vi "ADB-BlueTooth_2.vi"(11 "COM Port":refnum<visa-resource-name>="COM18") -> (0 "error out":errorcluster, 1 "Connectet":bool, 2 "AT CMD\n Status":bool, 3 "ADB PID":string, 4 "RSSI":i32)   [LabVIEW 2018]
panel:
  out "Progres Bar":u8(slide) scale=0.0..10.0
  out "ADB Data Monitor":string
  out "connect str1":string
  out "connect str2":string
  out "BLE-NINA-B1":string
  out "Mgg":string
  out "AT Cmd INI":string[][](array[string])=[["AT+CPWROFF", "", "+STARTUP"], ["AT+GMI", "u-blox", "OK"], ["AT+GMM", "NINA-B1", "OK"], ["ATI9", "NINA-B11X-5.0.0-011-0", "OK"], ["AT+GMR", "5.0.0-011", "OK"], ["AT+UMLA=1", "+UMLA:CCF95792B245", "OK"], ["AT+UBTLE=1", "", "OK"], ["AT&W", "", "OK"], ["AT+CPWROFF", "", "OK"], ["+AT+UBTLE?", "+UBTLE:1", "OK"]]
  out "AT-CMD/Date Monitor":string="\r\n"
  out "Status":T1(ring)
  out "Name":string
  out "SRS":string
  # "ADB-BlueTooth TEST"
  # "dbm"
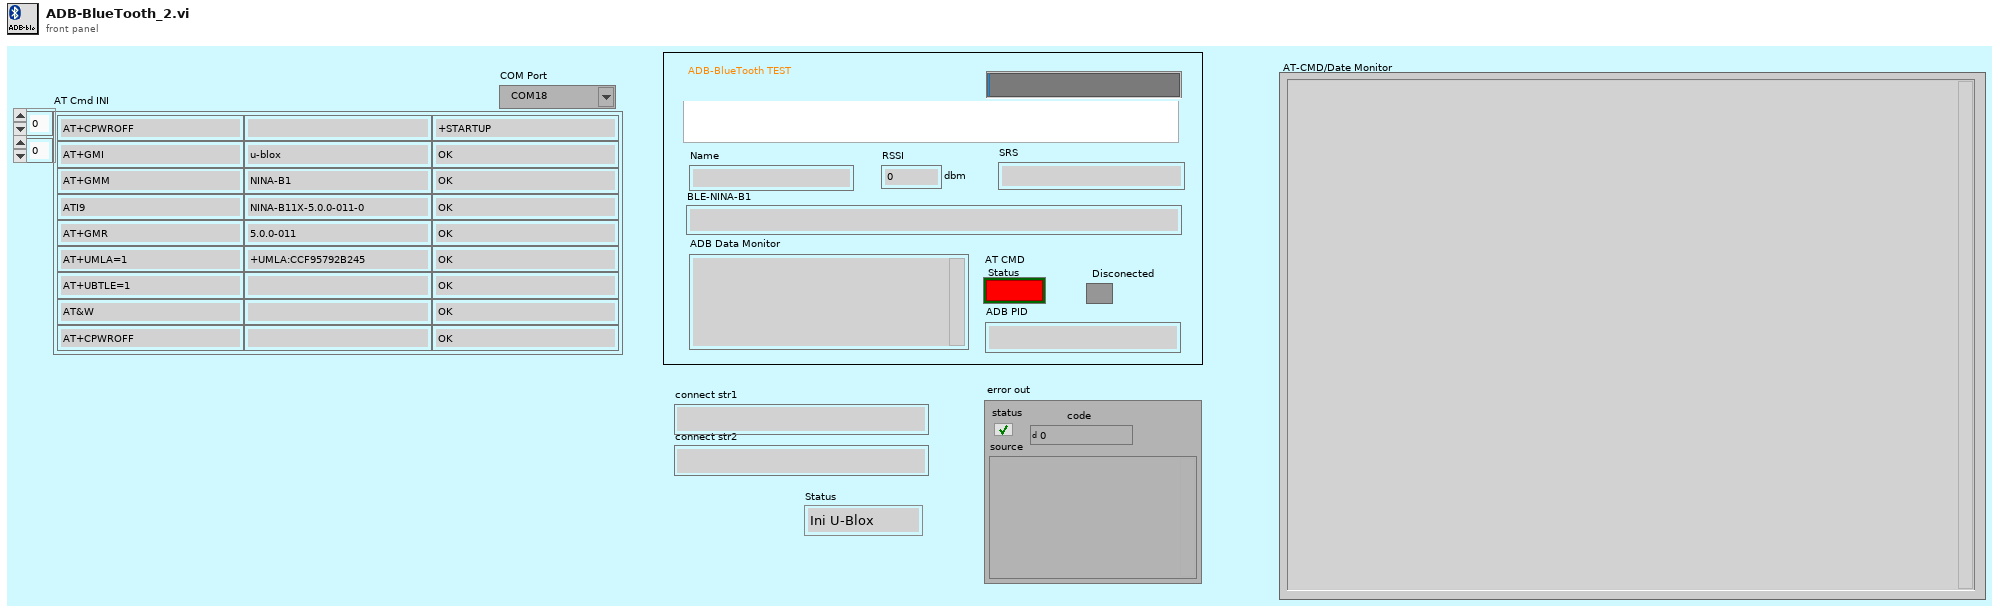
[diagram p1: front panel]
types:
  T1 = enum16{"Ini U-Blox", "Scan BLE Dev", "Connect to BLE", "Go-To DATA Mode", "Set BLE Admin", "BLE Red PID", "QUIT PAS/FALSE", "QUIT Err"}
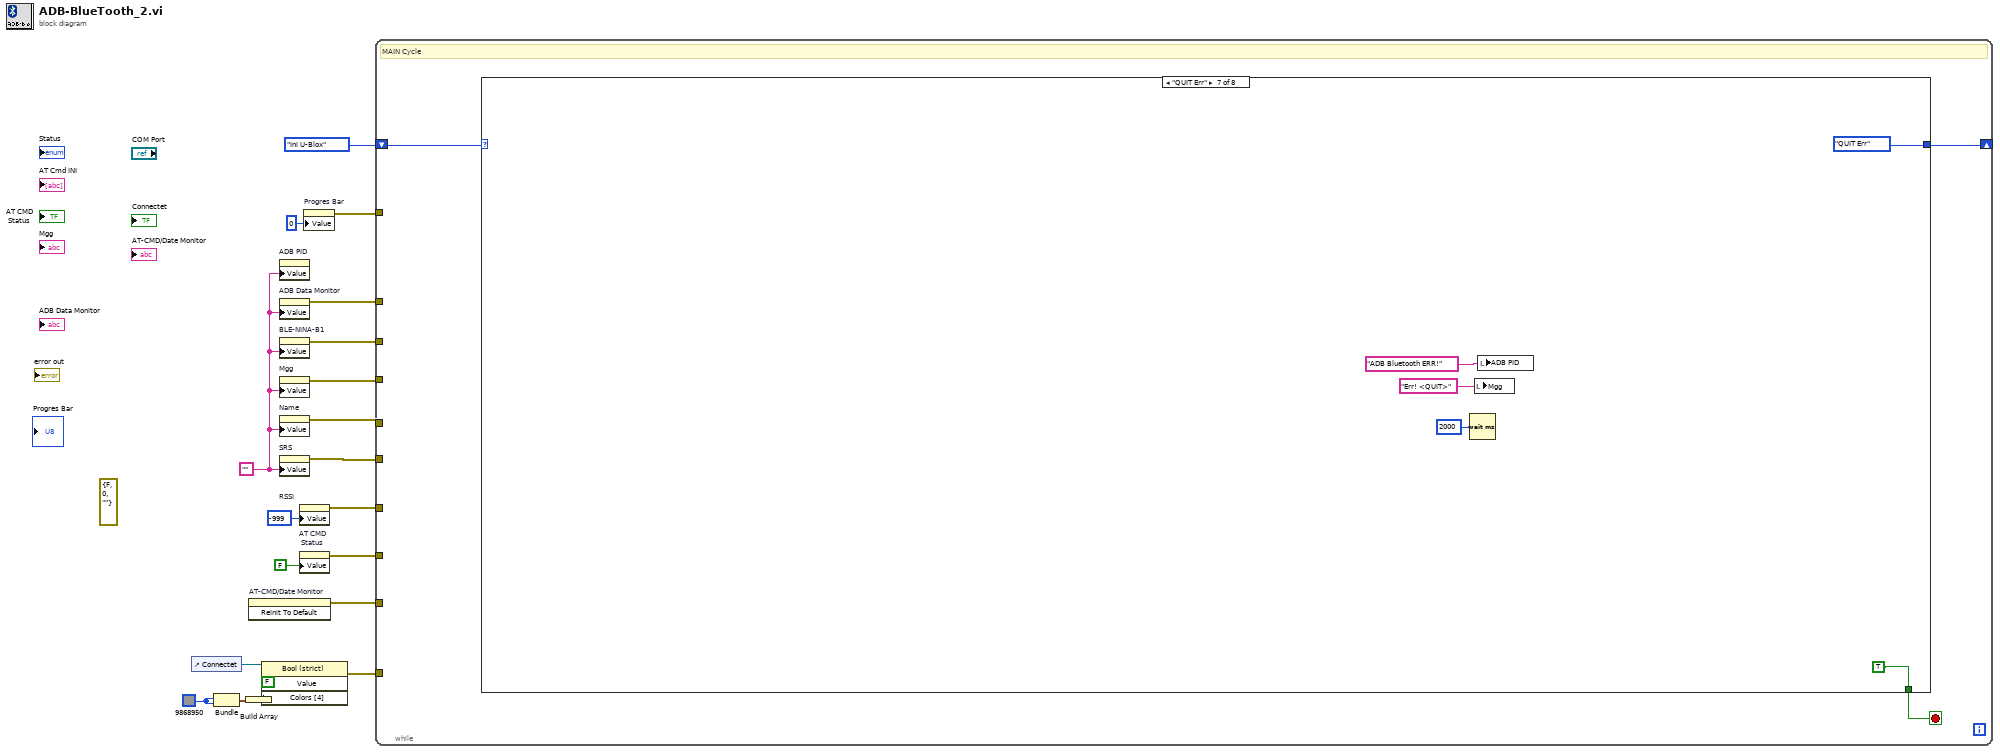
[diagram p0: block diagram]
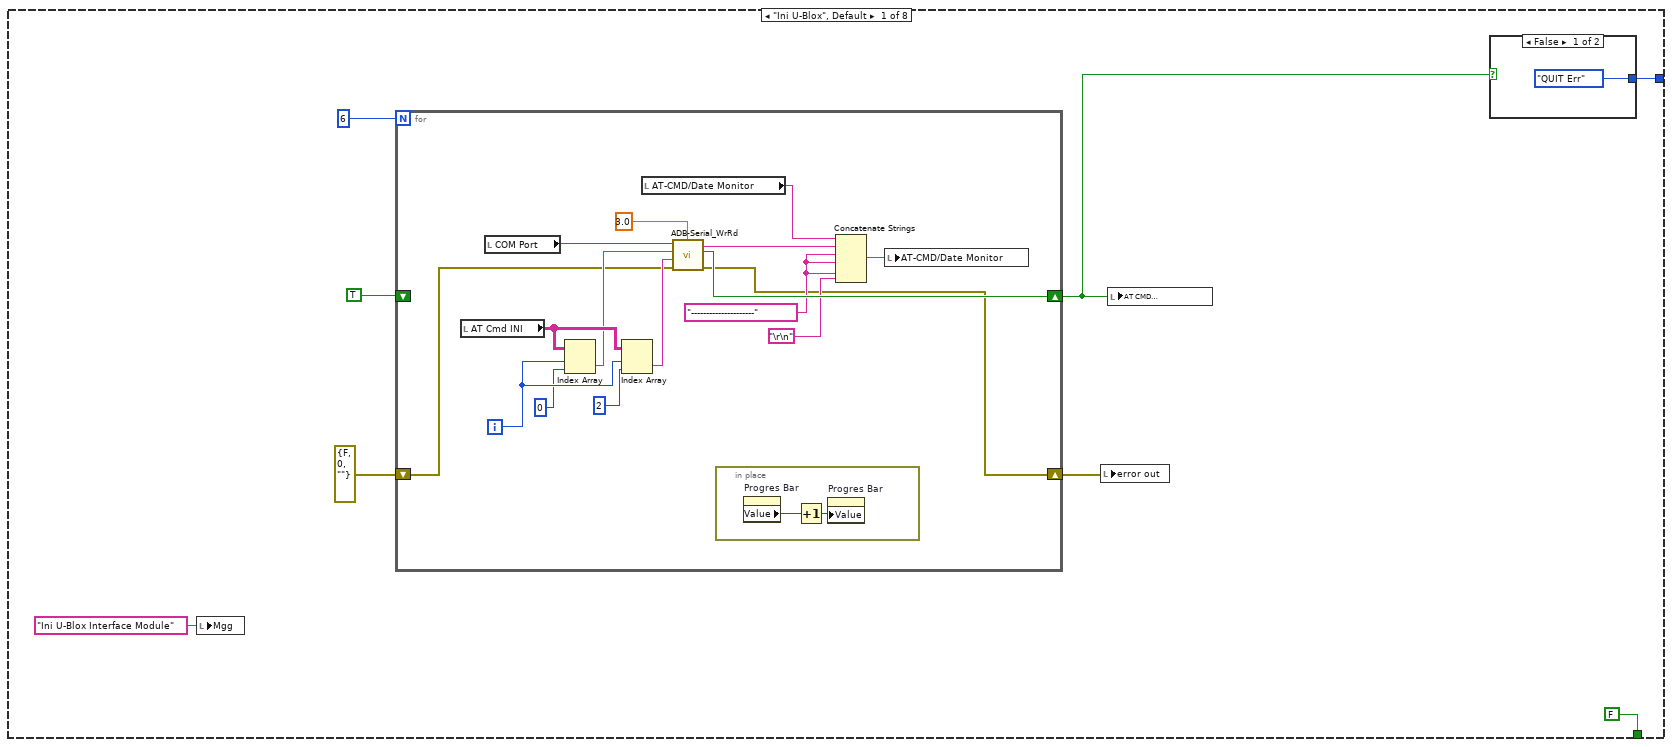
[diagram p2: hidden frame]
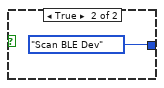
[diagram p3: hidden frame]
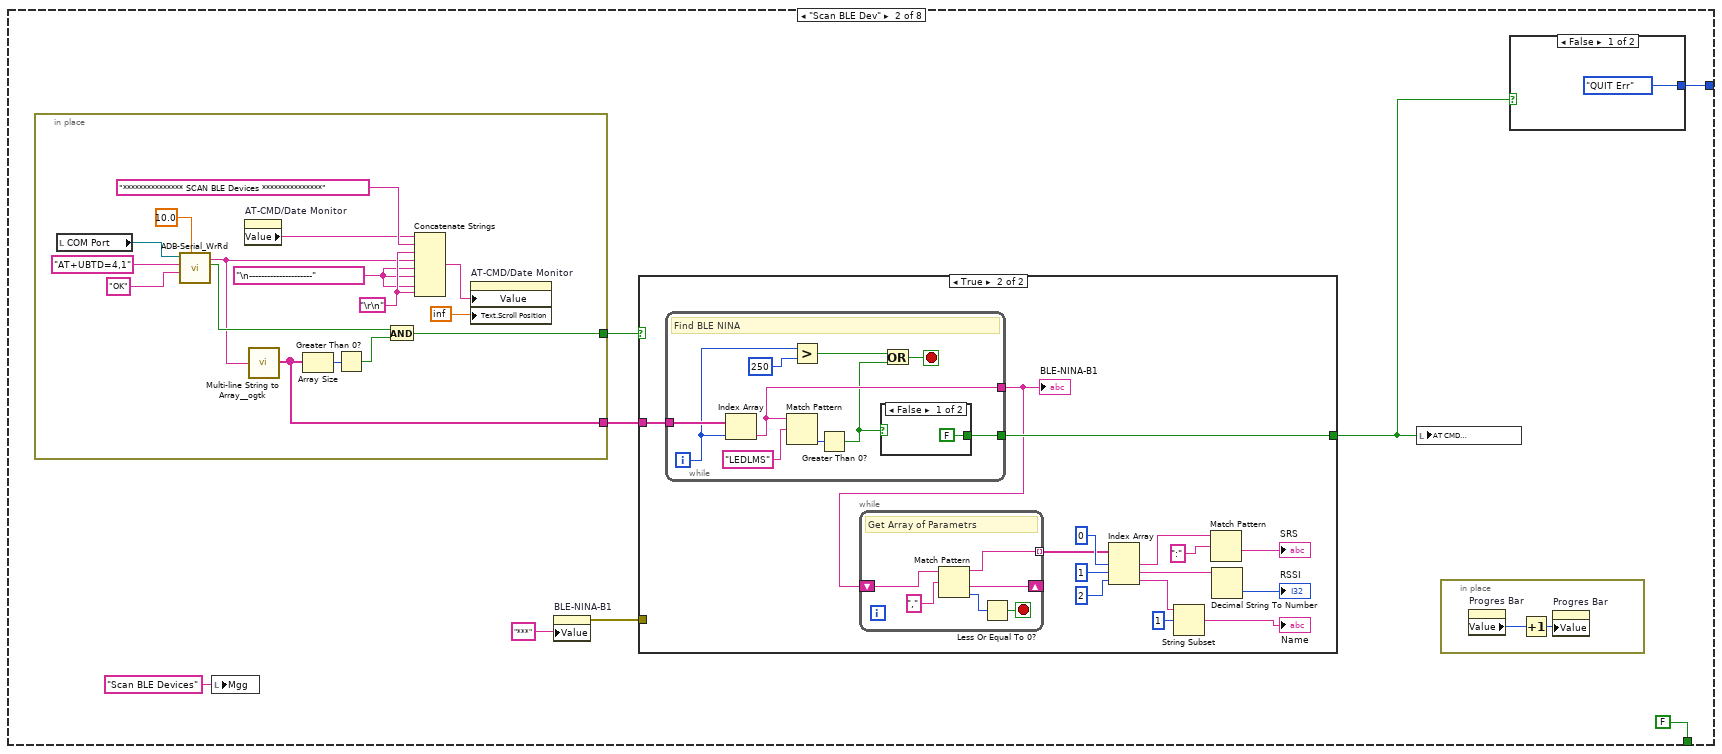
[diagram p4: hidden frame]
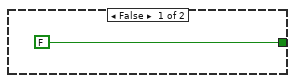
[diagram p5: hidden frame]
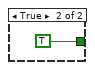
[diagram p6: hidden frame]
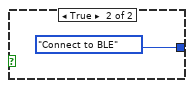
[diagram p7: hidden frame]
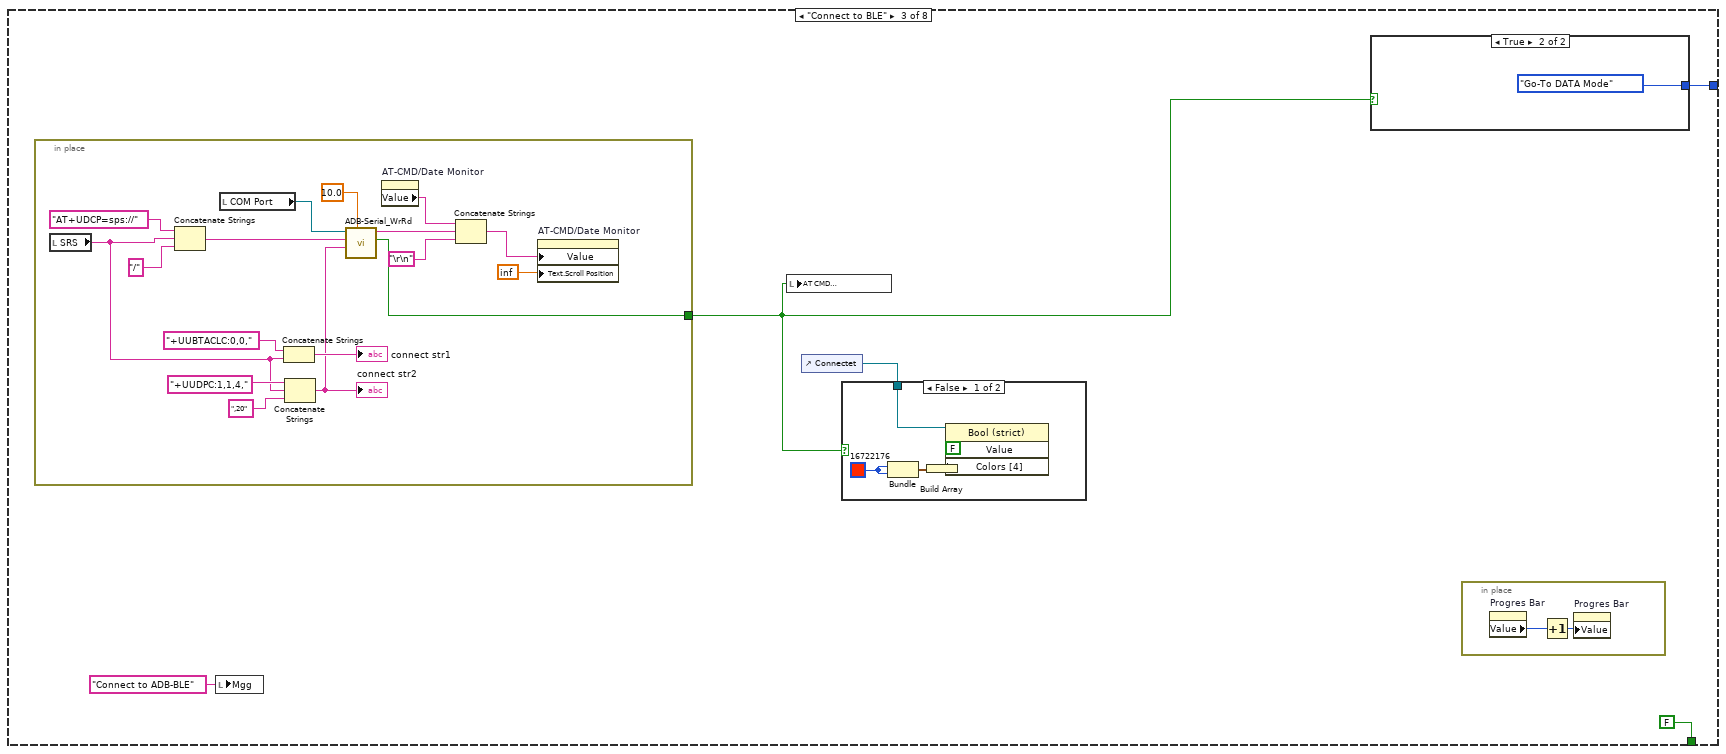
[diagram p8: hidden frame]
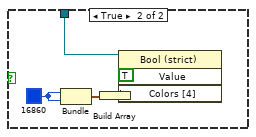
[diagram p9: hidden frame]
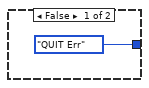
[diagram p10: hidden frame]
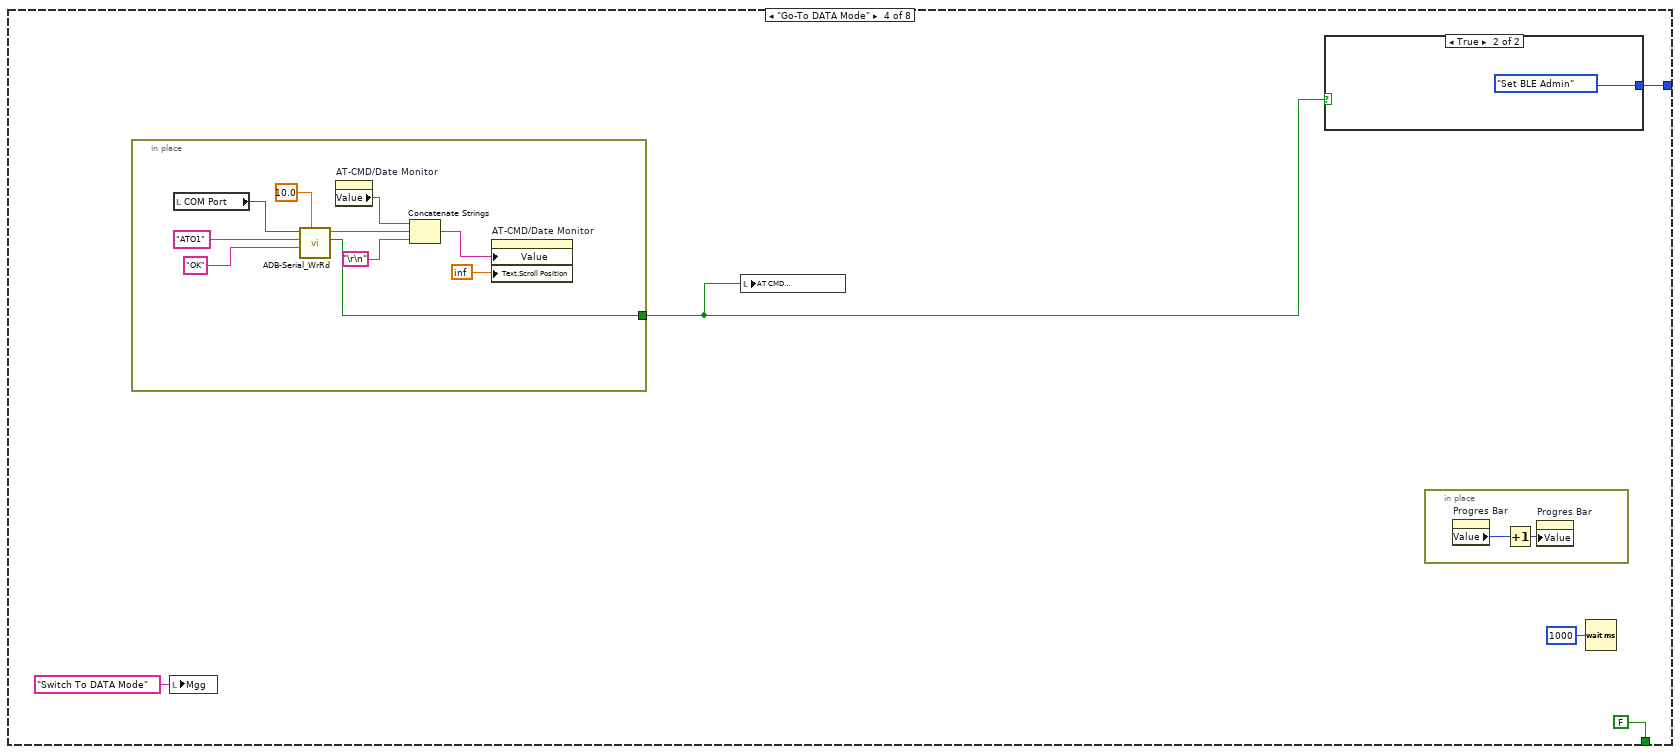
[diagram p11: hidden frame]
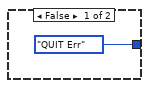
[diagram p12: hidden frame]
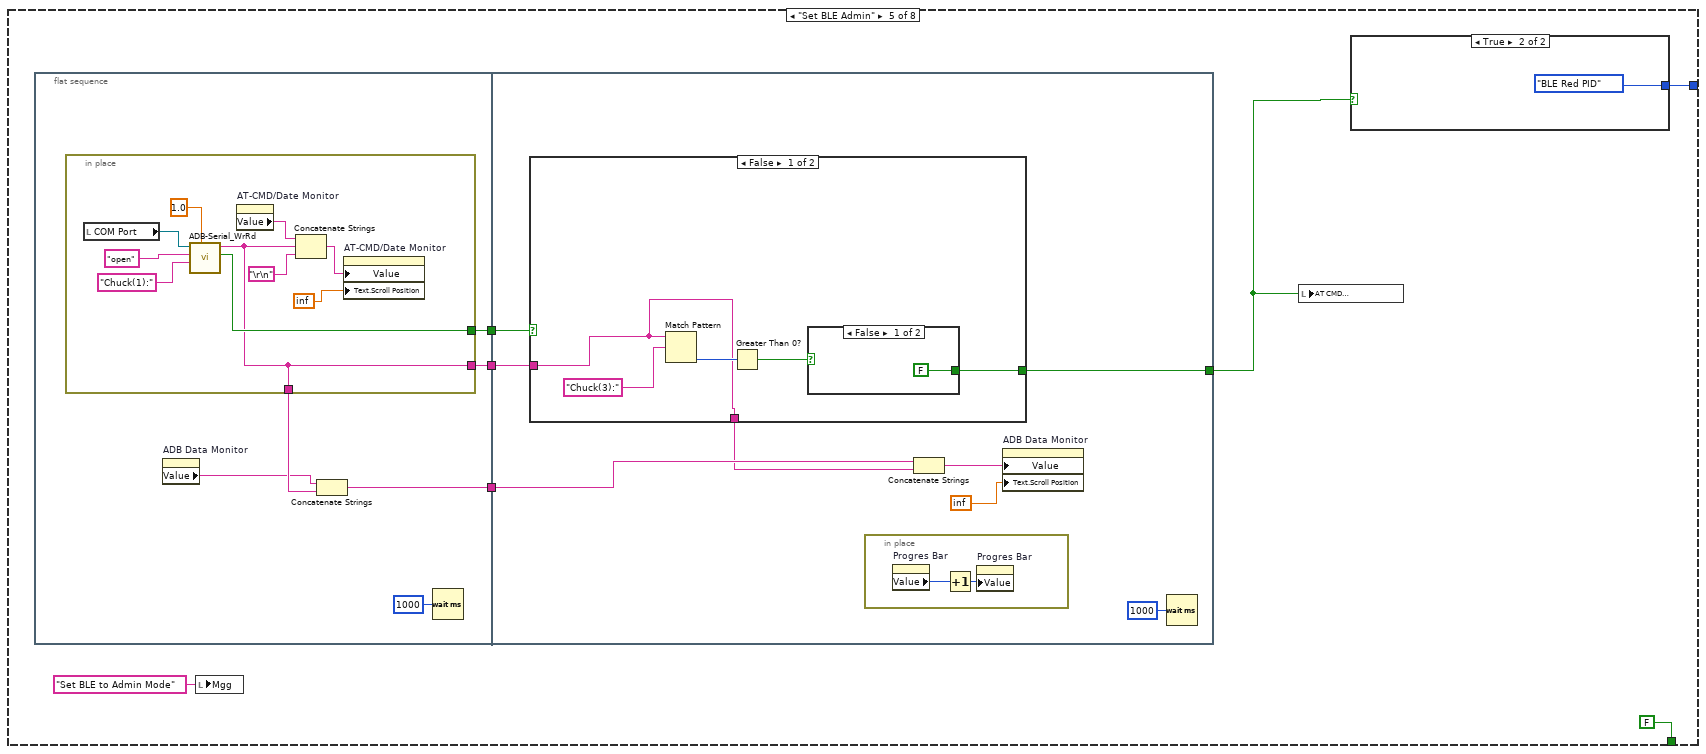
[diagram p13: hidden frame]
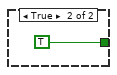
[diagram p14: hidden frame]
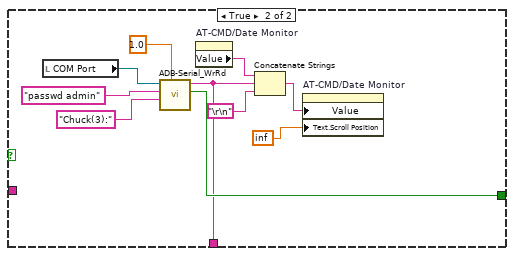
[diagram p15: hidden frame]
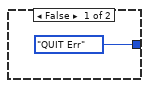
[diagram p16: hidden frame]
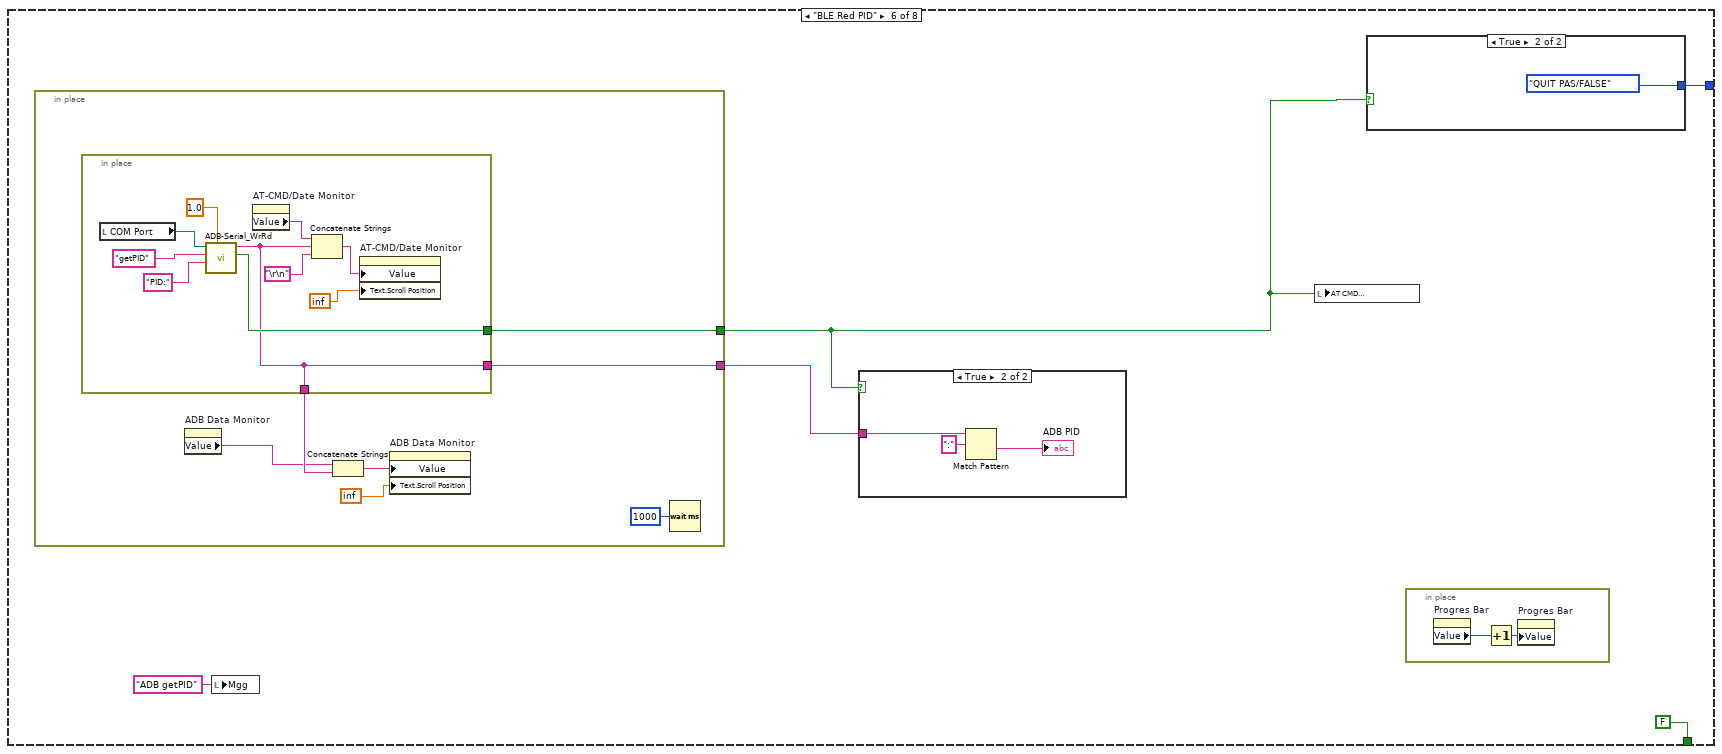
[diagram p17: hidden frame]
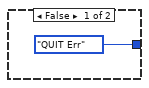
[diagram p19: hidden frame]
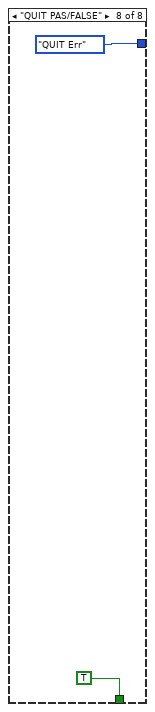
[diagram p20: hidden frame]
diagram:
  (unwired) errorcluster {"status"=FALSE, "code"=0, "source"=""} ("error constant")
  w8 = u32 9868950
  w3 = ""
  n1 = control-ref of="Connectet"() -> (w6:refnum<vi>)
  n2 = Bundle(w8, w8) -> (w10:cluster{u32, u32})  [unwired: 1 in]
  n3 = Build Array(w10) -> (w9:cluster{u32, u32}[])
  n4 = invoke on="AT-CMD/Date Monitor" class="Str" method="Reinit To Default"() -> (error out=w20:errorcluster)  [unwired: 3 in, 2 out]
  n5 = property on="Property Node" class="Bool (strict)"(reference=w6, "Value"=FALSE, "Colors [4]"=w9) -> (error out=w5:errorcluster)  [unwired: 1 in, 1 out]
  n6 = property on="ADB PID" class="Str"("Value"=w3) -> ()  [unwired: 2 in, 2 out]
  n7 = property on="ADB Data Monitor" class="Str"("Value"=w3) -> (error out=w4:errorcluster)  [unwired: 2 in, 1 out]
  n8 = property on="BLE-NINA-B1" class="Str"("Value"=w3) -> (error out=w12:errorcluster)  [unwired: 2 in, 1 out]
  n9 = property on="Mgg" class="Str"("Value"=w3) -> (error out=w13:errorcluster)  [unwired: 2 in, 1 out]
  n10 = property on="Name" class="Str"("Value"=w3) -> (error out=w14:errorcluster)  [unwired: 2 in, 1 out]
  n11 = property on="SRS" class="Str"("Value"=w3) -> (error out=w15:errorcluster)  [unwired: 2 in, 1 out]
  n12 = property on="RSSI" class="DigNum (strict)"("Value"=-999 ("RSSI")) -> (error out=w17:errorcluster)  [unwired: 2 in, 1 out]
  n13 = property on="AT CMD\n Status" class="Bool (strict)"("Value"=FALSE ("AT CMD Status")) -> (error out=w19:errorcluster)  [unwired: 2 in, 1 out]
  n14 = property on="Progres Bar" class="Slide (strict)"("Value"=u8 0 ("Progres Bar")) -> (error out=w2:errorcluster)  [unwired: 2 in, 1 out]
  n15 = while {
    shift-right: [w21] -> _
    shift-left: T1."Ini U-Blox" ("Status") -> [w22]
    tunnel: w20 -> [_]
    tunnel: w19 -> [_]
    tunnel: w17 -> [_]
    tunnel: w15 -> [_]
    tunnel: w14 -> [_]
    tunnel: w13 -> [_]
    tunnel: w12 -> [_]
    tunnel: w5 -> [_]
    tunnel: w4 -> [_]
    tunnel: w2 -> [_]
    stop <- w23 stop-if-true
    # "MAIN Cycle"
    n16 = case shown="\"QUIT Err\"" w22 {
      tunnel: [w31 w59 w116 w152 w173 w223 T1."QUIT Err" ("Status") T1."QUIT Err" ("Status")] -> w21
      tunnel: [FALSE FALSE FALSE FALSE FALSE FALSE TRUE TRUE] -> w23
      frame "Ini U-Blox", Default {
        n17 = local write "Mgg"("Ini U-Blox Interface Module" ("Mgg")) -> ()
        n18 = for {
          N: 6 -> [_]
          shift-right: [w48] -> w26
          shift-left: TRUE ("PASS") -> [_]
          shift-right: [w34] -> w24
          shift-left: errorcluster {"status"=FALSE, "code"=0, "source"=""} ("error constant") -> [w35]
          i -> [w46]
          w41 = "---------------------"
          n19 = local read "AT Cmd INI"() -> (w47:string[][])
          n20 = local read "COM Port"() -> (w38:refnum<visa-resource-name>)
          n21 = Index Array(array=w47, index (row)=w46, index (col)=0 ("disabled index (col)")) -> (element=w43:string)
          n22 = Index Array(array=w47, index (row)=w46, index (col)=2 ("disabled index (col)")) -> (element=w42:string)
          n23 = local read "AT-CMD/Date Monitor"() -> (w37:string)
          n24 = call "ADB-Serial_WrRd.vi"("Timeout(Sec)"=3.0, "error in (no error)"=w35, "PassString"=w42, "Command"=w43, "ComPort"=w38) -> ("error out"=w34:errorcluster, "PASS"=w48:bool, "received"=w49:string)  [unwired: 4 in]
          n25 = in-place {
            n26 = property on="Progres Bar" class="Slide (strict)"() -> ("Value"=w50:u8)  [unwired: 2 in, 2 out]
            n27 = Increment(x=w50) -> (x+1=w51:u8)
            n28 = property on="Progres Bar" class="Slide (strict)"("Value"=w51) -> ()  [unwired: 2 in, 2 out]
          }
          n29 = Concatenate Strings(w37, w49, w41, w41, w41, "\r\n") -> (w36:string)
          n30 = local write "AT-CMD/Date Monitor"(w36) -> ()
        }
        n31 = local write "error out"(w24) -> ()
        n32 = local write "AT CMD\n Status"(w26) -> ()
        n33 = case shown="False" w26 {
          tunnel: [T1."QUIT Err" ("Status") T1."Scan BLE Dev" ("Status")] -> w31
          frame False {
          }
          frame True {
          }
        }
      }
      frame "Scan BLE Dev" {
        n34 = in-place {
          in-place-border: [w63] -> w56
          in-place-border: [w62] -> w55
          w74 = "\r\n"
          w69 = "\n---------------------"
          n35 = local read "COM Port"() -> (w68:refnum<visa-resource-name>)
          n36 = call "ADB-Serial_WrRd.vi"("Timeout(Sec)"=10.0, "PassString"="OK", "Command"="AT+UBTD=4,1", "ComPort"=w68) -> ("PASS"=w77:bool, "received"=w64:string)  [unwired: 5 in, 1 out]
          n37 = property on="AT-CMD/Date Monitor" class="Str"() -> ("Value"=w67:string)  [unwired: 2 in, 2 out]
          n38 = call <userlib>:"Multi-line String to Array__ogtk.vi"("string"=w64) -> ("lines"=w62:string[])
          n39 = Array Size(array=w62) -> (size(s)=w73:i32)
          n40 = Greater Than 0?(x=w73) -> (x > 0?=w76:bool)
          n41 = And(x=w77, y=w76) -> (x .and. y?=w63:bool)
          n42 = Concatenate Strings(w67, "*************** SCAN BLE Devices ***************", w74, w64, w69, w69, w69, w74) -> (w66:string)
          n43 = property on="AT-CMD/Date Monitor" class="Str"("Value"=w66, "Text.Scroll Position"=inf) -> ()  [unwired: 2 in, 2 out]
        }
        n44 = local write "Mgg"("Scan BLE Devices" ("Mgg")) -> ()
        n45 = property on="BLE-NINA-B1" class="Str"("Value"="***" ("BLE-NINA")) -> (error out=w54:errorcluster)  [unwired: 2 in, 1 out]
        n46 = case shown="True" w56 {
          tunnel: w55 -> [_ w93]
          tunnel: [FALSE w92] -> w52
          tunnel: w54 -> [_ _]
          frame False {
          }
          frame True {
            n47 = while {
              tunnel: [w106] -> w91
              tunnel: w93 -> [w107]
              tunnel: [w100] -> w92
              i -> [w104]
              stop <- w103 stop-if-true
              # "Find BLE NINA"
              n48 = Index Array(array=w107, index=w104) -> (element=w106:string)
              n49 = Match Pattern(string=w106, regular expression="LEDLMS" ("element")) -> (offset past match=w109:i32)  [unwired: 1 in, 3 out]
              n50 = Greater?(x=w104, y=u16 250) -> (0:w102:bool)
              n51 = Greater Than 0?(x=w109) -> (x > 0?=w101:bool)
              n52 = case shown="False" w101 {
                tunnel: [FALSE TRUE] -> w100
                frame False {
                }
                frame True {
                }
              }
              n53 = Or(x=w102, y=w101) -> (x .or. y?=w103:bool)
            }
            "BLE-NINA-B1" <- w91
            n54 = while {
              shift-right: [w97] -> _
              shift-left: w91 -> [w98]
              tunnel: [w94] -> w87 mode=indexing
              stop <- w96 stop-if-true
              # "Get Array of Parametrs"
              n55 = Match Pattern(string=w98, regular expression=",") -> (before substring=w94:string, after substring=w97:string, offset past match=w95:i32)  [unwired: 1 in, 1 out]
              n56 = Less Or Equal To 0?(x=w95) -> (x <= 0?=w96:bool)
            }
            n57 = Index Array(array=w87, index #1=0 ("index"), index #2=1 ("index"), index #3=2 ("index")) -> (element #1=w85:string, element #2=w84:string, element #3=w81:string)
            n58 = String Subset(string=w81, offset (0)=1) -> (substring=→"Name":string)  [unwired: 1 in]
            n59 = Match Pattern(string=w85, regular expression=":") -> (after substring=→"SRS":string)  [unwired: 1 in, 3 out]
            n60 = Decimal String To Number(string=w84) -> (number=→"RSSI":i32)  [unwired: 2 in, 1 out]
          }
        }
        n61 = local write "AT CMD\n Status"(w52) -> ()
        n62 = in-place {
          n63 = property on="Progres Bar" class="Slide (strict)"() -> ("Value"=w60:u8)  [unwired: 2 in, 2 out]
          n64 = Increment(x=w60) -> (x+1=w61:u8)
          n65 = property on="Progres Bar" class="Slide (strict)"("Value"=w61) -> ()  [unwired: 2 in, 2 out]
        }
        n66 = case shown="False" w52 {
          tunnel: [T1."QUIT Err" ("Status") T1."Connect to BLE" ("Status")] -> w59
          frame False {
          }
          frame True {
          }
        }
      }
      frame "Connect to BLE" {
        n67 = in-place {
          in-place-border: [w131] -> w114
          n68 = local read "SRS"() -> (w137:string)
          n69 = Concatenate Strings("AT+UDCP=sps://" ("string"), w137, "/" ("string")) -> (w142:string)
          n70 = local read "COM Port"() -> (w146:refnum<visa-resource-name>)
          n71 = Concatenate Strings("+UUBTACLC:0,0,", w137) -> (→"connect str1":string)
          n72 = Concatenate Strings("+UUDPC:1,1,4,", w137, ",20") -> (w136:string)
          "connect str2" <- w136
          n73 = call "ADB-Serial_WrRd.vi"("Timeout(Sec)"=10.0, "PassString"=w136, "Command"=w142, "ComPort"=w146) -> ("PASS"=w131:bool, "received"=w134:string)  [unwired: 5 in, 1 out]
          n74 = property on="AT-CMD/Date Monitor" class="Str"() -> ("Value"=w135:string)  [unwired: 2 in, 2 out]
          n75 = Concatenate Strings(w135, w134, "\r\n") -> (w132:string)
          n76 = property on="AT-CMD/Date Monitor" class="Str"("Value"=w132, "Text.Scroll Position"=inf) -> ()  [unwired: 2 in, 2 out]
        }
        n77 = local write "Mgg"("Connect to ADB-BLE" ("Mgg")) -> ()
        n78 = local write "AT CMD\n Status"(w114) -> ()
        n79 = control-ref of="Connectet"() -> (w115:refnum<vi>)
        n80 = case shown="False" w114 {
          tunnel: w115 -> [w121 w126]
          frame False {
            w123 = u32 16722176
            n81 = Bundle(w123, w123) -> (w125:cluster{u32, u32})  [unwired: 1 in]
            n82 = Build Array(w125) -> (w124:cluster{u32, u32}[])
            n83 = property on="Property Node" class="Bool (strict)"(reference=w121, "Value"=FALSE, "Colors [4]"=w124) -> ()  [unwired: 1 in, 2 out]
          }
          frame True {
            w127 = u32 16860
            n84 = Bundle(w127, w127) -> (w130:cluster{u32, u32})  [unwired: 1 in]
            n85 = Build Array(w130) -> (w129:cluster{u32, u32}[])
            n86 = property on="Property Node" class="Bool (strict)"(reference=w126, "Value"=TRUE, "Colors [4]"=w129) -> ()  [unwired: 1 in, 2 out]
          }
        }
        n87 = case shown="True" w114 {
          tunnel: [T1."QUIT Err" ("Status") T1."Go-To DATA Mode" ("Status")] -> w116
          frame False {
          }
          frame True {
          }
        }
        n88 = in-place {
          n89 = property on="Progres Bar" class="Slide (strict)"() -> ("Value"=w119:u8)  [unwired: 2 in, 2 out]
          n90 = Increment(x=w119) -> (x+1=w120:u8)
          n91 = property on="Progres Bar" class="Slide (strict)"("Value"=w120) -> ()  [unwired: 2 in, 2 out]
        }
      }
      frame "Go-To DATA Mode" {
        n92 = in-place {
          in-place-border: [w159] -> w151
          n93 = local read "COM Port"() -> (w165:refnum<visa-resource-name>)
          n94 = call "ADB-Serial_WrRd.vi"("Timeout(Sec)"=10.0, "PassString"="OK" ("string"), "Command"="ATO1" ("string"), "ComPort"=w165) -> ("PASS"=w159:bool, "received"=w162:string)  [unwired: 5 in, 1 out]
          n95 = property on="AT-CMD/Date Monitor" class="Str"() -> ("Value"=w163:string)  [unwired: 2 in, 2 out]
          n96 = Concatenate Strings(w163, w162, "\r\n") -> (w160:string)
          n97 = property on="AT-CMD/Date Monitor" class="Str"("Value"=w160, "Text.Scroll Position"=inf) -> ()  [unwired: 2 in, 2 out]
        }
        n98 = local write "Mgg"("Switch To DATA Mode" ("Mgg")) -> ()
        n99 = local write "AT CMD\n Status"(w151) -> ()
        n100 = case shown="True" w151 {
          tunnel: [T1."QUIT Err" ("Status") T1."Set BLE Admin" ("Status")] -> w152
          frame False {
          }
          frame True {
          }
        }
        n101 = in-place {
          n102 = property on="Progres Bar" class="Slide (strict)"() -> ("Value"=w155:u8)  [unwired: 2 in, 2 out]
          n103 = Increment(x=w155) -> (x+1=w156:u8)
          n104 = property on="Progres Bar" class="Slide (strict)"("Value"=w156) -> ()  [unwired: 2 in, 2 out]
        }
        n105 = Wait (ms)(milliseconds to wait=u32 1000) -> ()  [unwired: 1 out]
      }
      frame "Set BLE Admin" {
        n106 = flat-sequence {
          tunnel: [w181] -> w172
          tunnel: [w180] -> w171
          tunnel: [w177] -> w169
          tunnel: w172 -> [w199]
          tunnel: w171 -> [w198]
          tunnel: [w196] -> w170
          tunnel: w169 -> [w195]
          frame #0 {
            n107 = in-place {
              in-place-border: [w186] -> w181
              in-place-border: [w182] -> w180
              in-place-border: [w182] -> w178
              n108 = local read "COM Port"() -> (w190:refnum<visa-resource-name>)
              n109 = call "ADB-Serial_WrRd.vi"("Timeout(Sec)"=1.0, "PassString"="Chuck(1):" ("string"), "Command"="open" ("string"), "ComPort"=w190) -> ("PASS"=w186:bool, "received"=w182:string)  [unwired: 5 in, 1 out]
              n110 = property on="AT-CMD/Date Monitor" class="Str"() -> ("Value"=w189:string)  [unwired: 2 in, 2 out]
              n111 = Concatenate Strings(w189, w182, "\r\n") -> (w187:string)
              n112 = property on="AT-CMD/Date Monitor" class="Str"("Value"=w187, "Text.Scroll Position"=inf) -> ()  [unwired: 2 in, 2 out]
            }
            n113 = property on="ADB Data Monitor" class="Str"() -> ("Value"=w176:string)  [unwired: 2 in, 2 out]
            n114 = Concatenate Strings(w176, w178) -> (w177:string)
            n115 = Wait (ms)(milliseconds to wait=u32 1000) -> ()  [unwired: 1 out]
          }
          frame #1 {
            n116 = case shown="False" w199 {
              tunnel: w198 -> [w202 _]
              tunnel: [w203 w210] -> w196
              tunnel: [w202 w209] -> w194
              frame False {
                n117 = Match Pattern(string=w202, regular expression="Chuck(3):" ("string")) -> (offset past match=w205:i32)  [unwired: 1 in, 3 out]
                n118 = Greater Than 0?(x=w205) -> (x > 0?=w204:bool)
                n119 = case shown="False" w204 {
                  tunnel: [FALSE TRUE] -> w203
                  frame False {
                  }
                  frame True {
                  }
                }
              }
              frame True {
                n120 = local read "COM Port"() -> (w212:refnum<visa-resource-name>)
                n121 = call "ADB-Serial_WrRd.vi"("Timeout(Sec)"=1.0, "PassString"="Chuck(3):" ("string"), "Command"="passwd admin" ("string"), "ComPort"=w212) -> ("PASS"=w210:bool, "received"=w209:string)  [unwired: 5 in, 1 out]
                n122 = property on="AT-CMD/Date Monitor" class="Str"() -> ("Value"=w213:string)  [unwired: 2 in, 2 out]
                n123 = Concatenate Strings(w213, w209, "\r\n") -> (w215:string)
                n124 = property on="AT-CMD/Date Monitor" class="Str"("Value"=w215, "Text.Scroll Position"=inf) -> ()  [unwired: 2 in, 2 out]
              }
            }
            n125 = in-place {
              n126 = property on="Progres Bar" class="Slide (strict)"() -> ("Value"=w200:u8)  [unwired: 2 in, 2 out]
              n127 = Increment(x=w200) -> (x+1=w201:u8)
              n128 = property on="Progres Bar" class="Slide (strict)"("Value"=w201) -> ()  [unwired: 2 in, 2 out]
            }
            n129 = Concatenate Strings(w195, w194) -> (w193:string)
            n130 = property on="ADB Data Monitor" class="Str"("Value"=w193, "Text.Scroll Position"=inf) -> ()  [unwired: 2 in, 2 out]
            n131 = Wait (ms)(milliseconds to wait=u32 1000) -> ()  [unwired: 1 out]
          }
        }
        n132 = local write "Mgg"("Set BLE to Admin Mode" ("Mgg")) -> ()
        n133 = local write "AT CMD\n Status"(w170) -> ()
        n134 = case shown="True" w170 {
          tunnel: [T1."QUIT Err" ("Status") T1."BLE Red PID" ("Status")] -> w173
          frame False {
          }
          frame True {
          }
        }
      }
      frame "BLE Red PID" {
        n135 = in-place {
          in-place-border: [w237] -> w222
          in-place-border: [w231] -> w221
          n136 = in-place {
            in-place-border: [w242] -> w237
            in-place-border: [w238] -> w231
            in-place-border: [w238] -> w236
            n137 = local read "COM Port"() -> (w246:refnum<visa-resource-name>)
            n138 = call "ADB-Serial_WrRd.vi"("Timeout(Sec)"=1.0, "PassString"="PID:" ("string"), "Command"="getPID" ("string"), "ComPort"=w246) -> ("PASS"=w242:bool, "received"=w238:string)  [unwired: 5 in, 1 out]
            n139 = property on="AT-CMD/Date Monitor" class="Str"() -> ("Value"=w245:string)  [unwired: 2 in, 2 out]
            n140 = Concatenate Strings(w245, w238, "\r\n") -> (w243:string)
            n141 = property on="AT-CMD/Date Monitor" class="Str"("Value"=w243, "Text.Scroll Position"=inf) -> ()  [unwired: 2 in, 2 out]
          }
          n142 = property on="ADB Data Monitor" class="Str"() -> ("Value"=w235:string)  [unwired: 2 in, 2 out]
          n143 = Concatenate Strings(w235, w236) -> (w234:string)
          n144 = property on="ADB Data Monitor" class="Str"("Value"=w234, "Text.Scroll Position"=inf) -> ()  [unwired: 2 in, 2 out]
          n145 = Wait (ms)(milliseconds to wait=u32 1000) -> ()  [unwired: 1 out]
        }
        n146 = local write "Mgg"("ADB getPID" ("Mgg")) -> ()
        n147 = case shown="True" w222 {
          tunnel: w221 -> [_ w230]
          frame False {
          }
          frame True {
            n148 = Match Pattern(string=w230, regular expression=":") -> (after substring=→"ADB PID":string)  [unwired: 1 in, 3 out]
          }
        }
        n149 = local write "AT CMD\n Status"(w222) -> ()
        n150 = case shown="True" w222 {
          tunnel: [T1."QUIT Err" ("Status") T1."QUIT PAS/FALSE" ("Status")] -> w223
          frame False {
          }
          frame True {
          }
        }
        n151 = in-place {
          n152 = property on="Progres Bar" class="Slide (strict)"() -> ("Value"=w226:u8)  [unwired: 2 in, 2 out]
          n153 = Increment(x=w226) -> (x+1=w227:u8)
          n154 = property on="Progres Bar" class="Slide (strict)"("Value"=w227) -> ()  [unwired: 2 in, 2 out]
        }
      }
      frame "QUIT Err" {
        n155 = Wait (ms)(milliseconds to wait=u32 2000) -> ()  [unwired: 1 out]
        n156 = local write "Mgg"("Err! <QUIT>" ("Mgg")) -> ()
        n157 = local write "ADB PID"("ADB Bluetooth ERR!") -> ()
      }
      frame "QUIT PAS/FALSE" {
      }
    }
  }
